vi "Create Enum Data Clusters.vi"(8 "error in (no error)":errorcluster, 9 "Generate_SerializationHelper":bool, 10 "Enum parameters":T1[](array[typedef]), 11 "Library in":refnum<vi>) -> (0 "error out":errorcluster, 3 "Library out":refnum<vi>)   [LabVIEW 2019, in "gRPC Template Creation Utility.lvlib"]
uses:
  gRPC Template Creation Utility.lvlib
  TypeDefs/Enum Metadata (Scripting).ctl
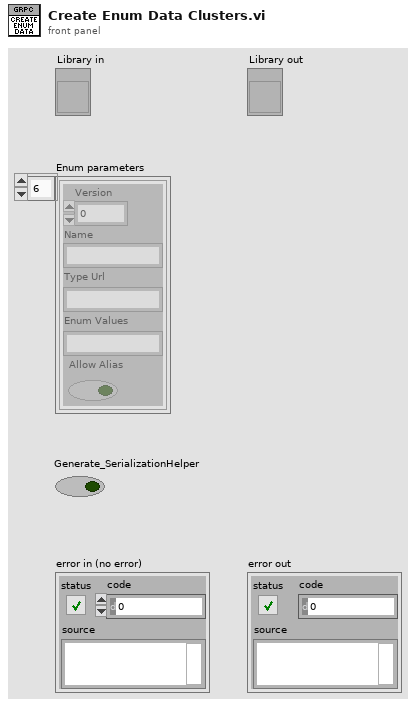
[diagram p1: front panel]
types:
  T1 = typedef "gRPC Template Creation Utility.lvlib/Enum Metadata (Scripting).ctl" = cluster{"Version":i32, "Name":string, "Type Url":string, "Enum Values":string, "Allow Alias":bool}
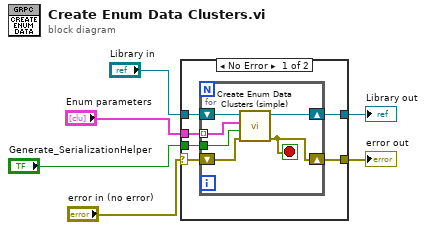
[diagram p0: block diagram]
diagram:
  n1 = case shown="No Error" "error in (no error)" {
    selector: "error in (no error)" -> [w8 w19]
    tunnel: "Enum parameters" -> [w12 _]
    tunnel: [w10 w20] -> w5
    tunnel: [w11 w19] -> w4
    tunnel: "Library in" -> [w9 w20]
    tunnel: "Generate_SerializationHelper" -> [w7 _]
    frame No Error {
      n2 = for {
        shift-right: [w16] -> w10
        shift-left: w9 -> [w18]
        shift-right: [w15] -> w11
        shift-left: w8 -> [w17]
        tunnel: w12 -> [w14] mode=indexing
        tunnel: w7 -> [w13]
        stop <- w15 stop-if-true
        n3 = call "Create Enum Data Clusters (simple).vi"("error in (no error)"=w17, "Generate_SerializationHelper"=w13, "Enum Metadata"=w14, "Library"=w18) -> ("error out"=w15:errorcluster, "Library"=w16:refnum<vi>)  [unwired: 6 in]
      }
    }
    frame Error {
    }
  }
  "Library out" <- w5
  "error out" <- w4
